vi "AprilTagFieldLayout_SetOrigin.vi"(9 "OriginPosition":T7, 11 "in AprilTagFieldLayout":T1={"AprilTagMap"={}, "FieldLength"=0.0, "FieldWidth"=0.0, "OriginPosition "=enum."kBlueAllianceWallRightSide,", "OriginPose3d"={"Translation3d"={"X"=0.0, "Y"=0.0, "Z"=0.0}, "Rotation3d"={"Q_quaternion"={"R"=1.0, "V"=[0.0, 0.0, 0.0]}}}} {"OriginPose3d"."Translation3d"."Z" format="%14.3f"; "OriginPose3d"."Translation3d"."Y" format="%14.3f"; "OriginPose3d"."Translation3d"."X" format="%14.3f"}) -> (1 "OriginPose3d":T3={"Translation3d"={"X"=0.0, "Y"=0.0, "Z"=0.0}, "Rotation3d"={"Q_quaternion"={"R"=1.0, "V"=[0.0, 0.0, 0.0]}}} {"Translation3d"."Z" format="%14.3f"; "Translation3d"."Y" format="%14.3f"; "Translation3d"."X" format="%14.3f"}, 3 "out AprilTagFieldLayout":T1={"AprilTagMap"={}, "FieldLength"=0.0, "FieldWidth"=0.0, "OriginPosition "=enum."kBlueAllianceWallRightSide,", "OriginPose3d"={"Translation3d"={"X"=0.0, "Y"=0.0, "Z"=0.0}, "Rotation3d"={"Q_quaternion"={"R"=1.0, "V"=[0.0, 0.0, 0.0]}}}} {"OriginPose3d"."Translation3d"."Z" format="%14.3f"; "OriginPose3d"."Translation3d"."Y" format="%14.3f"; "OriginPose3d"."Translation3d"."X" format="%14.3f"})   [LabVIEW 2019, in "Trajectory_Library.lvlib"]
doc: "Sets the origin based on a predefined enumeration of coordinate frame origins. The origins are calculated from the field dimensions.\n\nThis transforms the Pose3d objects returned by {@link #getTagPose(int)} to return the correct pose relative to a predefined coordinate frame.\n\nInputs:\n -- in AprilTagFieldLayout -- AprilTagFieldLayout -- Input field data cluster.\n -- OriginPosition -- enum -- The predefined origin\n\nOutputs:\n -- out AprilTagFieldLayout -- AprilTagFieldLayout -- Modified field data cluster\n -- OriginPosition3d -- Pose3d -- Position of the origin."
uses:
  Trajectory_Library.lvlib
  TypeDef/AprilTagFieldLayout.ctl
  TypeDef/AprilTag.ctl
  TypeDef/POSE3D.ctl
  TypeDef/TRANSLATION3D.ctl
  TypeDef/ROTATION3D.ctl
  TypeDef/QUATERNION.ctl
  Enum/AprilTagFieldLayoutOrignPosition_ENUM.ctl
  Quaternion_New.vi
  Translation3d_Create_Default.vi
  Rotation3d_Create_Default.vi
  Quaternion_New_Default.vi
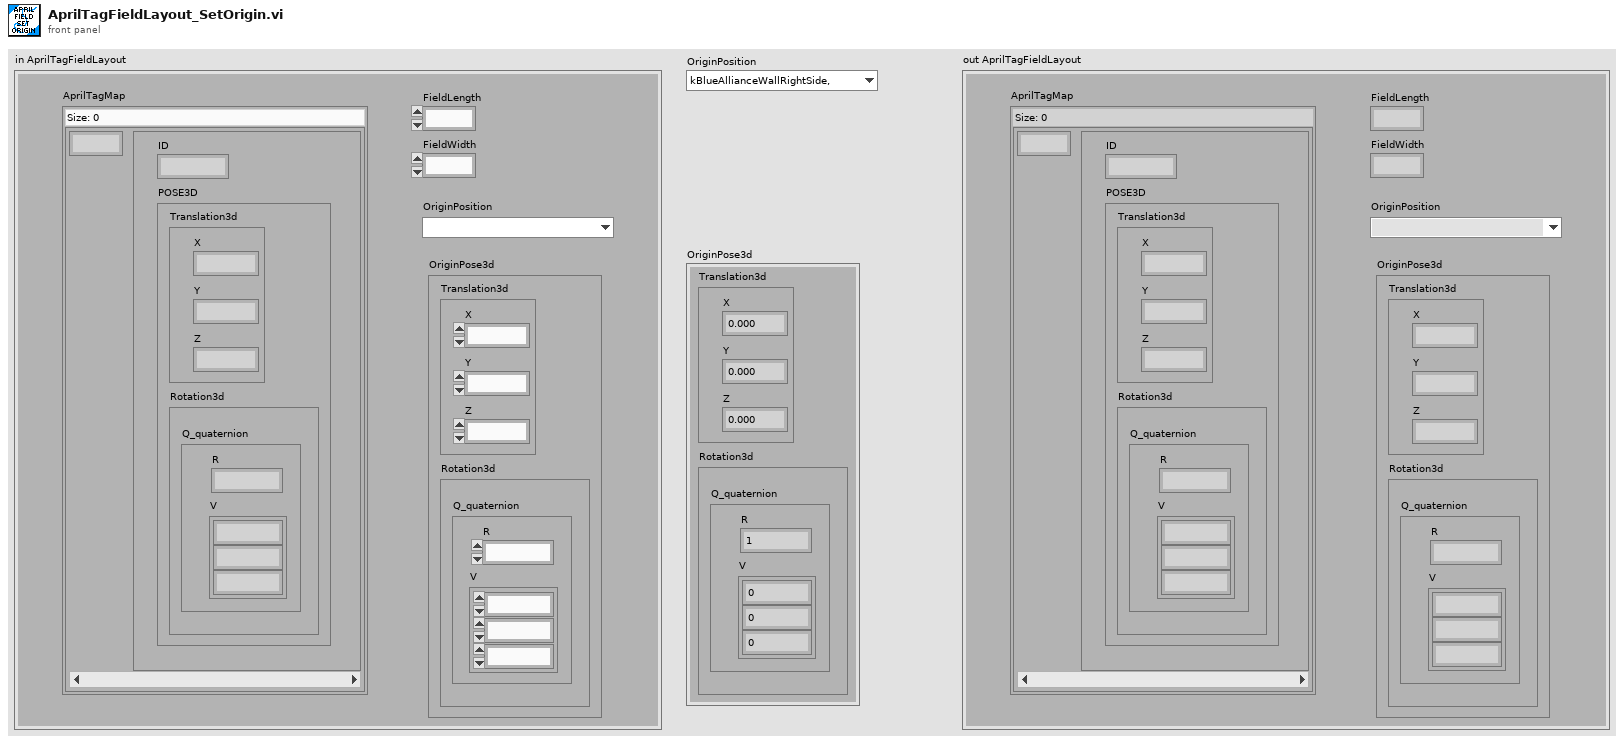
[diagram p1: front panel]
types:
  T1 = typedef "Trajectory_Library.lvlib/AprilTagFieldLayout.ctl" = cluster{"AprilTagMap":map{i32, T2}, "FieldLength":dbl, "FieldWidth":dbl, "OriginPosition ":T7, "OriginPose3d":T3}
  T2 = typedef "Trajectory_Library.lvlib/AprilTag.ctl" = cluster{"ID":i32, "POSE3D":T3}
  T3 = typedef "Trajectory_Library.lvlib/POSE3D.ctl" = cluster{"Translation3d":T4, "Rotation3d":T5}
  T4 = typedef "Trajectory_Library.lvlib/TRANSLATION3D.ctl" = cluster{"X":dbl, "Y":dbl, "Z":dbl}
  T5 = typedef "Trajectory_Library.lvlib/ROTATION3D.ctl" = cluster{"Q_quaternion":T6}
  T6 = typedef "Trajectory_Library.lvlib/QUATERNION.ctl" = cluster{"R":dbl, "V":dbl[]}
  T7 = typedef "Trajectory_Library.lvlib/AprilTagFieldLayoutOrignPosition_ENUM.ctl" = enum16{"kBlueAllianceWallRightSide,", "kRedAllianceWallRightSide,"}
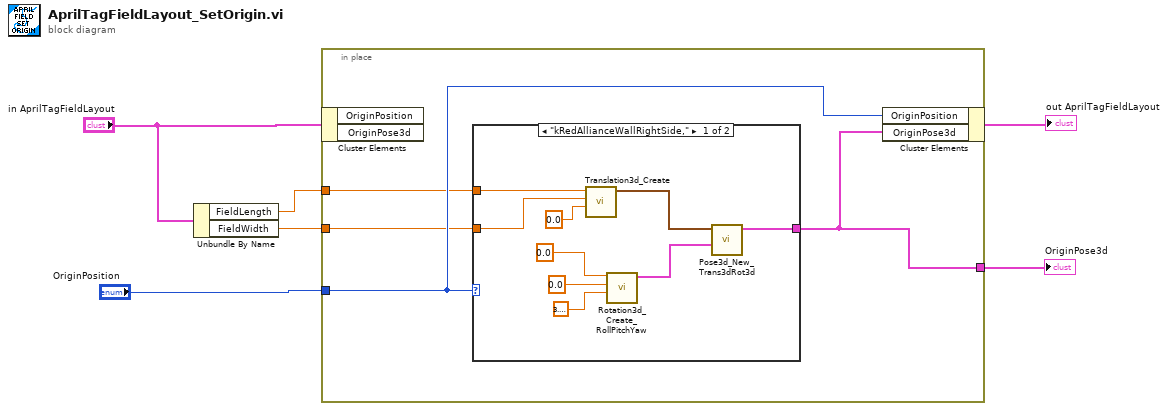
[diagram p0: block diagram]
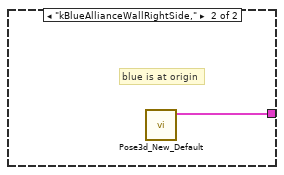
[diagram p2: hidden frame]
diagram:
  n1 = Unbundle By Name("in AprilTagFieldLayout") -> ("FieldLength"=w2:dbl, "FieldWidth"=w3:dbl)
  n2 = in-place {
    in-place-border: "OriginPosition" -> [w10]
    in-place-border: w2 -> [w9]
    in-place-border: w3 -> [w8]
    in-place-border: [w7] -> w1
    n3 = in-place-cluster #1("in AprilTagFieldLayout") -> ()  [unwired: 2 out]
    n4 = case shown="\"kRedAllianceWallRightSide,\"" w10 {
      tunnel: [w19 w20] -> w7
      tunnel: w9 -> [w17 _]
      tunnel: w8 -> [w12 _]
      frame "kRedAllianceWallRightSide," {
        n5 = call "Translation3d_Create.vi"("Z"=0.0, "Y"=w12, "X"=w17) -> ("TRANSLATION3D"=w18:T4)  [unwired: 8 in]
        n6 = call "Rotation3d_Create_RollPitchYaw.vi"("Yaw"=3.141592653589793, "Pitch"=0.0, "Roll"=0.0) -> ("Rotation3d"=w16:T5)  [unwired: 8 in]
        n7 = call "Pose3d_New_Trans3dRot3d.vi"("Rotation3d"=w16, "Translation3d"=w18) -> ("outPose3d"=w19:T3)  [unwired: 9 in]
      }
      frame "kBlueAllianceWallRightSide," {
        # "blue is at origin"
        n8 = call "Pose3d_New_Default.vi"() -> ("outPose3d"=w20:T3)  [unwired: 11 in]
      }
    }
    n9 = in-place-cluster #1("OriginPosition"=w10, "OriginPose3d"=w7) -> (→"out AprilTagFieldLayout":T1)
  }
  "OriginPose3d" <- w1
